vi "Handle Errors.vi"(8 "error in":errorcluster, 11 "tCRD in":refnum<class "tCRD.lvclass">) -> (0 "error out":errorcluster, 2 "errors":errorcluster[](array[cluster]), 3 "tCRD out":refnum<class "tCRD.lvclass">)   [LabVIEW 2015, in "tCRD.lvclass"]
uses:
  tCRD.lvclass
  Reusable/CRDS/Main/CRDS.lvclass
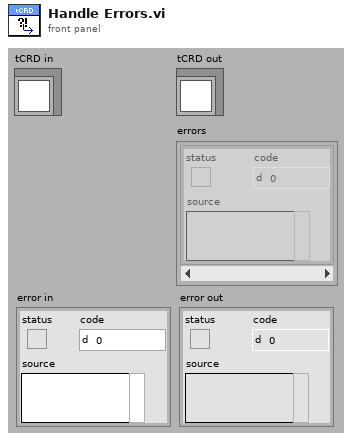
[diagram p1: front panel]
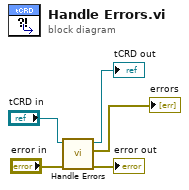
[diagram p0: block diagram]
diagram:
  n1 = call-parent "Handle Errors.vi"("error in"="error in", "Instrument in"="tCRD in") -> ("error out"=→"error out":errorcluster, "errors"=→"errors":errorcluster[], "Instrument out"=→"tCRD out":refnum<class "tCRD.lvclass">)  [unwired: 7 in]
